vi "ni272x Write Resistance nChan 1Samp.vi"(8 "error in (no error)":errorcluster, 9 "requested resistances (ohms)":dbl[](array[numeric]), 10 "resistor channels":string[](array[string]), 11 "instrument handle":T1) -> (0 "error out":errorcluster, 1 "coerced resistance (ohms)":dbl[](array[numeric]), 3 "instrument handle out":T1)   [LabVIEW 2017, in "NI 272x Resistive Simulation Custom Device Engine.lvlib"]
doc: "Sets the resistance on the <B> resistor channel</B> on a device initialized by the ni272x Initialize Session VI.\n\n<B>NOTE:</B> Writing a resistance value to a channel internally configures the bank resistance, but does not connect the bank to either front connector. To connect the internal resistance to either front connector, use the"
uses:
  <instrlib>/ni272xReferenceVIs/ni272xReferenceVIs.llb/ni272x Reference.ctl
  <instrlib>/ni272xReferenceVIs/ni272xReferenceVIs.llb/ni272x Attribute ID Device U8.ctl
  <instrlib>/ni272xReferenceVIs/ni272xReferenceVIs.llb/ni272x Attribute ID Channel Single.ctl
  <instrlib>/ni272xReferenceVIs/ni272xReferenceVIs.llb/ni272x Relay Control Action.ctl
  <instrlib>/ni272xReferenceVIs/ni272xReferenceVIs.llb/ni272x Error Code Offsets.ctl
  <instrlib>/ni272xReferenceVIs/ni272xReferenceVIs.llb/ni272x Set Attribute Channel Single.vi
  <instrlib>/ni272xReferenceVIs/ni272xReferenceVIs.llb/ni272x Relay Control Multiple.vi
  <instrlib>/ni272xReferenceVIs/ni272xReferenceVIs.llb/ni272x Get Attribute Device U8.vi
  <instrlib>/ni272xReferenceVIs/ni272xReferenceVIs.llb/ni272x Parse Channel String.vi
  <instrlib>/ni272xReferenceVIs/ni272xReferenceVIs.llb/ni272x Error Check Initialized.vi
  NI 272x Resistive Simulation Custom Device Engine.lvlib
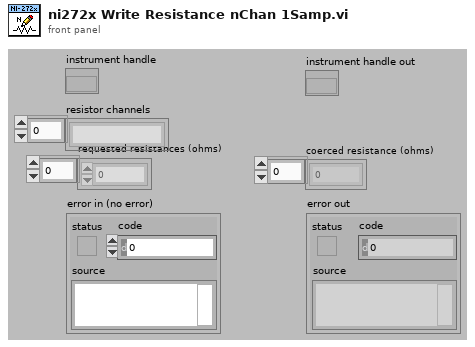
[diagram p1: front panel]
types:
  T1 = typedef "ni272x Reference.ctl" = refnum<k20>
  T2 = typedef "ni272x Relay Control Action.ctl" = enum16{"Open Relay", "Close Relay"}
  T3 = typedef "ni272x Attribute ID Channel Single.ctl" = enum16{"Minimum Resistance", "Maximum Resistance", "Resistance"}
  T4 = typedef "ni272x Attribute ID Device U8.ctl" = enum16{"Number of Banks", "Number of Channels", "Banks per Channel", "Bits per Bank"}
  T5 = typedef "ni272x Error Code Offsets.ctl" = enum16{"NI_272x_ERROR_BASE", "NI_272x_ERROR_DEVICE_NOT_SUPPORTED", "NI_272x_ERROR_DEVICE_NOT_INITIALIZED", "NI_272x_ERROR_BANK_NUMBER_OUT_OF_RANGE", "NI_272x_ERROR_CHANNEL_NUMBER_OUT_OF_RANGE", "NI_272x_ERROR_INVALID_ATTRIBUTE_ID", "NI_272x_ERROR_REQUESTED_RESISTANCE_OUT_OF_RANGE", "NI_272x_ERROR_BANKS_NOT_ADJACENT", "NI_272x_ERROR_CHANNELS_NOT_ADJACENT", "NI_272x_ERROR_INVALID_REFNUM", "NI_272x_ERROR_ATTRIBUTE_READ_ONLY", "NI_272x_ERROR_RESISTANCE_VALUE_NOT_SET", "NI_272x_ERROR_INVALID_BITS_PER_CHANNEL", "NI_272x_ERROR_INVALID_CONFIGURATION_DATA", "NI_272x_ERROR_INVALID_CONFIGURATION_FILE_VERSION", "NI_272x_ERROR_CONFIGURATION_FILE_CORRUPT", "NI_272x_INTERNAL_ERROR_INVALID_SEMAPHORE", "NI_272x_ERROR_PARSING_CHANNEL_STRING", "NI_272x_ERROR_PARSING_BANK_STRING", "NI_272x_ERROR_BANK_ALREADY_CONNECTED", "NI_272x_ERROR_CHANNEL_BANK_ALREADY_CONNECTED", "NI_272x_ERROR_BANK_ALREADY_CONNECTED_TO_DMM", "NI_272x_ERROR_ADJACENT_BANK_ALREADY_CONNECTED_TO_DUT", "NI_272x_ERROR_ADJACENT_BANK_STATUS_NOT_CONSISTENT"}
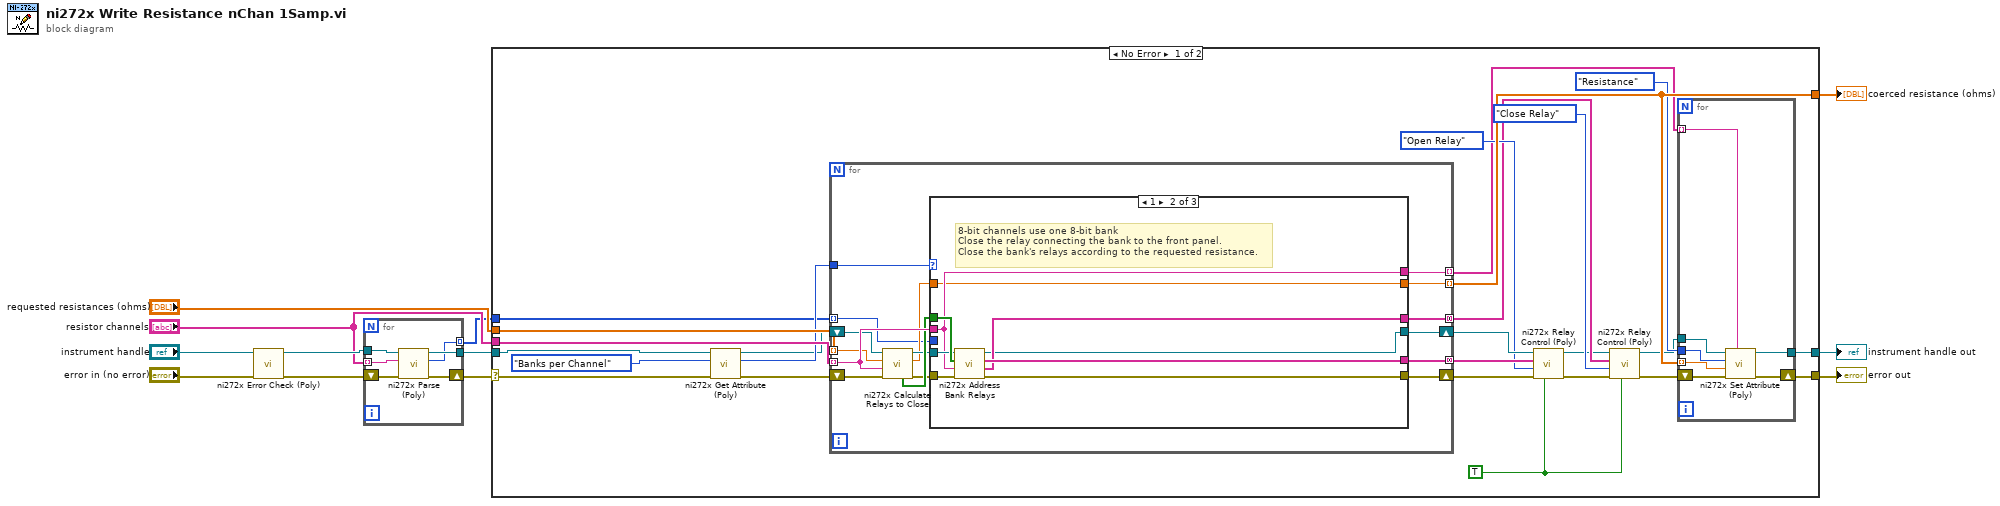
[diagram p0: block diagram]
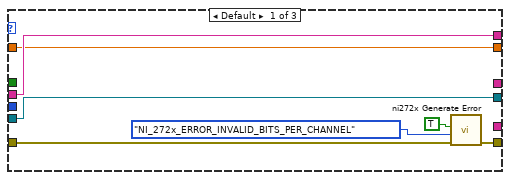
[diagram p2: hidden frame]
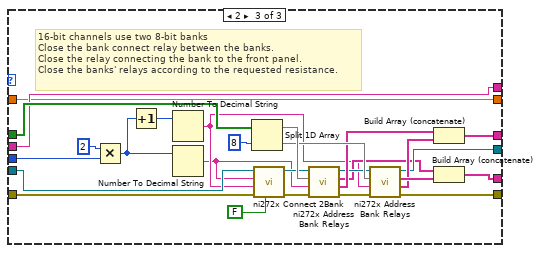
[diagram p3: hidden frame]
diagram:
  n1 = call-poly <instrlib>:"ni272x Error Check (Poly).vi"("error in (no error)"="error in (no error)", "instrument handle"="instrument handle") -> ("error out"=w4:errorcluster, "instrument handle out"=w6:T1)  [unwired: 8 out]
  n2 = for {
    tunnel: "resistor channels" -> [w14] mode=indexing
    tunnel: [w13] -> w1 mode=indexing
    shift-right: [w15] -> w3
    shift-left: w4 -> [w16]
    tunnel: w6 -> [w18]
    tunnel: [w17] -> w5
    n3 = call-poly <instrlib>:"ni272x Parse (Poly).vi"("error in (no error)"=w16, "channel string"=w14, "instrument handle"=w18) -> ("error out"=w15:errorcluster, "channel number"=w13:i32, "instrument handle out"=w17:T1)  [unwired: 6 out]
  }
  n4 = case shown="No Error" w3 {
    selector: w3 -> [w38 w112]
    tunnel: [w43 w112] -> w12
    tunnel: w5 -> [w39 w111]
    tunnel: [w42 w111] -> w11
    tunnel: "resistor channels" -> [w41 _]
    tunnel: "requested resistances (ohms)" -> [w37 w110]
    tunnel: [w36 w110] -> w8
    tunnel: w1 -> [w23 _]
    frame No Error {
      w29 = TRUE ("wait for settling")
      n5 = call-poly <instrlib>:"ni272x Get Attribute (Poly).vi"("error in (no error)"=w38, "attribute ID device u8"=ni272x_Attribute_ID_Device_U8."Banks per Channel" ("272x Attribute ID_Device_U8"), "instrument handle"=w39) -> ("error out"=w24:errorcluster, "device u8 attribute value"=w26:u8, "instrument handle out"=w25:T1)  [unwired: 6 out]
      n6 = for {
        tunnel: w41 -> [w59] mode=indexing
        tunnel: w37 -> [w58] mode=indexing
        tunnel: [w57] -> w36 mode=indexing
        tunnel: [w52] -> w33 mode=concatenating
        tunnel: [w50] -> w30 mode=concatenating
        tunnel: [w49] -> w27 mode=indexing
        tunnel: w26 -> [w47]
        tunnel: w23 -> [w44] mode=indexing
        shift-right: [w53] -> w34
        shift-left: w25 -> [w46]
        shift-right: [w51] -> w31
        shift-left: w24 -> [w45]
        n7 = call <instrlib>:"ni272x Calculate Relays to Close.vi"("error in (no error)"=w45, "resistor channel"=w59, "requested resistance (ohms)"=w58, "instrument handle"=w46) -> ("error out"=w54:errorcluster, "coerced resistance (ohms)"=w48:sgl, "instrument handle out"=w55:T1, "relays to close"=w56:bool[])  [unwired: 4 out]
        n8 = case shown="1" w47 {
          tunnel: w56 -> [_ w75 w102]
          tunnel: w59 -> [w61 w68 w80]
          tunnel: [_ w74 w84] -> w52
          tunnel: [_ w73 w83] -> w50
          tunnel: w54 -> [w63 w72 w89]
          tunnel: [w62 w71 w94] -> w51
          tunnel: w55 -> [w66 w70 w93]
          tunnel: [w66 w69 w85] -> w53
          tunnel: [w61 w68 w80] -> w49
          tunnel: w48 -> [w60 w67 w79]
          tunnel: [w60 w67 w79] -> w57
          tunnel: w44 -> [_ _ w78]
          frame Default {
            n9 = call <instrlib>:"ni272x Generate Error.vi"("error in (no error)"=w63, "272x error code"=ni272x_Error_Code_Offsets."NI_272x_ERROR_INVALID_BITS_PER_CHANNEL" ("272x Error Code"), "generate error?"=TRUE ("Generate Error?")) -> ("error out"=w62:errorcluster)  [unwired: 1 in, 7 out]
          }
          frame 1 {
            # "8-bit channels use one 8-bit bank\nClose the relay connecting the bank to the front panel.\nClose the bank's relays according to the requested resistance."
            n10 = call <instrlib>:"ni272x Address Bank Relays.vi"("error in (no error)"=w72, "resistor bank"=w68, "relays to close"=w75, "instrument handle"=w70) -> ("error out"=w71:errorcluster, "relays to close"=w73:string[], "relays to open"=w74:string[], "instrument handle out"=w69:T1)  [unwired: 4 out]
          }
          frame 2 {
            # "16-bit channels use two 8-bit banks\nClose the bank connect relay between the banks.\nClose the relay connecting the bank to the front panel.\nClose the banks' relays according to the requested resistance."
            n11 = Multiply(x=u8 2 ("y"), y=w78) -> (x*y=w91:i32)
            n12 = Increment(x=w91) -> (x+1=w90:i32)
            n13 = Number To Decimal String(number=w90) -> (decimal integer string=w77:string)  [unwired: 1 out]
            n14 = Number To Decimal String(number=w91) -> (decimal integer string=w76:string)  [unwired: 1 out]
            n15 = Split 1D Array(array=w102, index=8) -> (first subarray=w100:bool[], second subarray=w99:bool[])
            n16 = call <instrlib>:"ni272x Connect 2Bank.vi"("wait for settling (T)"=FALSE, "error in (no error)"=w89, "resistor bank N+1"=w77, "resistor bank N"=w76, "instrument handle"=w93) -> ("error out"=w88:errorcluster, "instrument handle out"=w87:T1)  [unwired: 5 out]
            n17 = call <instrlib>:"ni272x Address Bank Relays.vi"("error in (no error)"=w88, "resistor bank"=w76, "relays to close"=w100, "instrument handle"=w87) -> ("error out"=w98:errorcluster, "relays to close"=w96:string[], "relays to open"=w81:string[], "instrument handle out"=w86:T1)  [unwired: 4 out]
            n18 = call <instrlib>:"ni272x Address Bank Relays.vi"("error in (no error)"=w98, "resistor bank"=w77, "relays to close"=w99, "instrument handle"=w86) -> ("error out"=w94:errorcluster, "relays to close"=w95:string[], "relays to open"=w97:string[], "instrument handle out"=w85:T1)  [unwired: 4 out]
            n19 = Build Array (concatenate)(w96, w95) -> (w83:string[])
            n20 = Build Array (concatenate)(w81, w97) -> (w84:string[])
          }
        }
      }
      n21 = call-poly <instrlib>:"ni272x Relay Control (Poly).vi"("wait for settling (T)"=w29, "error in (no error)"=w31, "relay action"=ni272x_Relay_Control_Action."Open Relay" ("Relay Action"), "relay names"=w33, "instrument handle"=w34) -> ("error out"=w21:errorcluster, "instrument handle out"=w22:T1)  [unwired: 5 out]
      n22 = call-poly <instrlib>:"ni272x Relay Control (Poly).vi"("wait for settling (T)"=w29, "error in (no error)"=w21, "relay action"=ni272x_Relay_Control_Action."Close Relay" ("Relay Action"), "relay names"=w30, "instrument handle"=w22) -> ("error out"=w19:errorcluster, "instrument handle out"=w20:T1)  [unwired: 5 out]
      n23 = for {
        tunnel: w36 -> [w107] mode=indexing
        tunnel: ni272x_Attribute_ID_Channel_Single."Resistance" ("272x Attribute ID_Channel_Single") -> [w106]
        tunnel: w27 -> [w105] mode=indexing
        shift-right: [w109] -> w43
        shift-left: w19 -> [w103]
        tunnel: w20 -> [w104]
        tunnel: [w108] -> w42
        n24 = call-poly <instrlib>:"ni272x Set Attribute (Poly).vi"("resistor channel"=w105, "error in (no error)"=w103, "channel single attribute value"=w107, "attribute ID channel single"=w106, "instrument handle"=w104) -> ("error out"=w109:errorcluster, "instrument handle out"=w108:T1)  [unwired: 5 out]
      }
    }
    frame Error {
    }
  }
  "error out" <- w12
  "instrument handle out" <- w11
  "coerced resistance (ohms)" <- w8
